vi "GetSplittersWidths.vi"(8 "error in (no error)":errorcluster, 11 "Splitters":T1) -> (0 "error out":errorcluster, 3 "Splitters Widths":T2)   [LabVIEW 2022 SP3, in "PentaPanesLibrary.lvlib" / "PentaPanes.lvclass"]
uses:
  PentaPanes.lvclass
  SplittersWidthCluster.ctl
  SplittersCluster.ctl
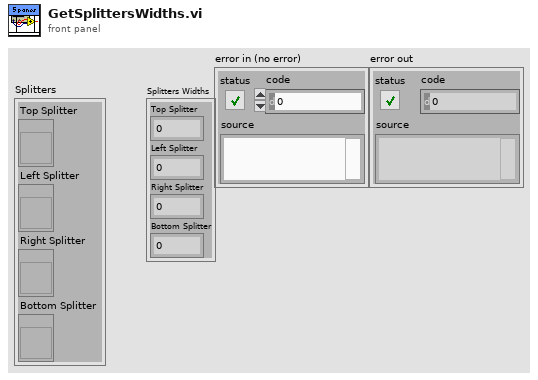
[diagram p1: front panel]
types:
  T1 = typedef "PentaPanesLibrary.lvlib/PentaPanes.lvclass/SplittersCluster.ctl" = cluster{"Top Splitter":refnum<vi>, "Left Splitter":refnum<vi>, "Right Splitter":refnum<vi>, "Bottom Splitter":refnum<vi>}
  T2 = typedef "PentaPanesLibrary.lvlib/PentaPanes.lvclass/SplittersWidthCluster.ctl" = cluster{"Top Splitter":i32, "Left Splitter":i32, "Right Splitter":i32, "Bottom Splitter":i32}
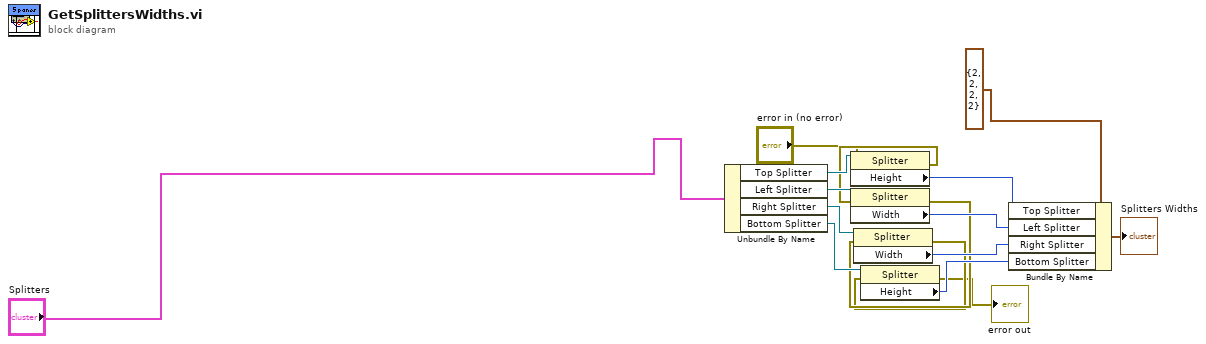
[diagram p0: block diagram]
diagram:
  n1 = Unbundle By Name("Splitters") -> ("Top Splitter"=w7:refnum<vi>, "Left Splitter"=w10:refnum<vi>, "Right Splitter"=w11:refnum<vi>, "Bottom Splitter"=w9:refnum<vi>)
  n2 = property class="Splitter"(reference=w7, error in="error in (no error)") -> (error out=w5:errorcluster, "Height"=w8:u32)  [unwired: 1 out]
  n3 = property class="Splitter"(reference=w10, error in=w5) -> (error out=w4:errorcluster, "Width"=w12:u32)  [unwired: 1 out]
  n4 = property class="Splitter"(reference=w11, error in=w4) -> (error out=w3:errorcluster, "Width"=w13:u32)  [unwired: 1 out]
  n5 = property class="Splitter"(reference=w9, error in=w3) -> (error out=→"error out":errorcluster, "Height"=w14:u32)  [unwired: 1 out]
  n6 = Bundle By Name(cluster=T2 {"Top Splitter"=2, "Left Splitter"=2, "Right Splitter"=2, "Bottom Splitter"=2} ("Splitters Widths"), "Top Splitter"=w8, "Left Splitter"=w12, "Right Splitter"=w13, "Bottom Splitter"=w14) -> (→"Splitters Widths":T2)
